vi "List Users.vi"(8 "error in (no error)":errorcluster, 11 "I Authentication Provider in":refnum<class "I Authentication Provider.lvclass">) -> (0 "error out":errorcluster, 2 "Users":string[](array[string]), 3 "I Authentication Provider out":refnum<class "I Authentication Provider.lvclass">)   [LabVIEW 2026, in "I Authentication Provider.lvclass"]
uses:
  I Authentication Provider.lvclass
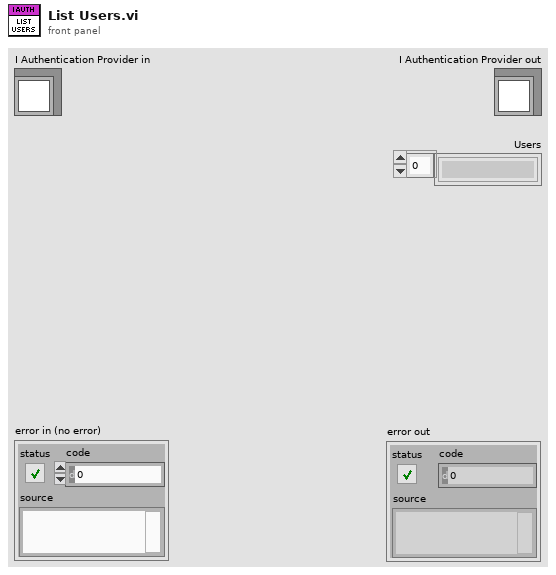
[diagram p1: front panel]
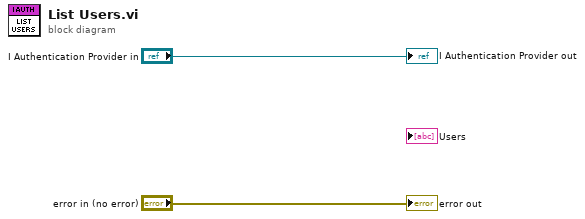
[diagram p0: block diagram]
diagram:
  "error out" <- "error in (no error)"
  "I Authentication Provider out" <- "I Authentication Provider in"
